vi "Get Stage Limits.vi"(0 "Notifier Names":string[](array[string]), 2 "Notifier Name":string, 7 "Stage Limits":T1[](array[typedef]), 11 "Limits Loaded?":bool) -> (4 "Limits":dbl[][](array[numeric]), 15 "Use Limits?":bool)   [LabVIEW 2016]
uses:
  Stages Limits Type Defs/Stage Limits.ctl
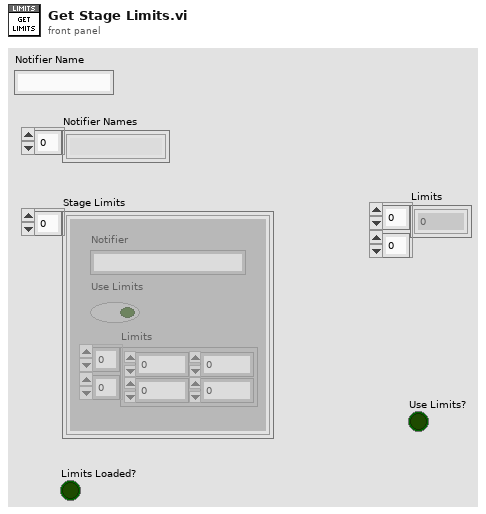
[diagram p1: front panel]
types:
  T1 = typedef "Stage Limits.ctl" = cluster{"Notifier":string, "Use Limits":bool, "Limits":dbl[][]}
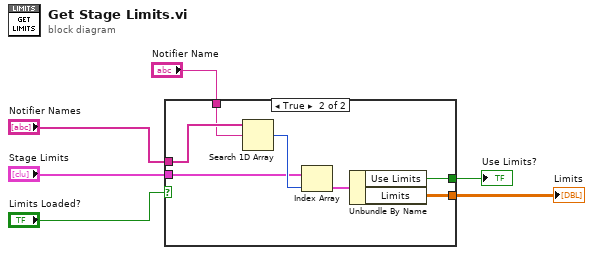
[diagram p0: block diagram]
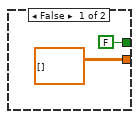
[diagram p2: hidden frame]
diagram:
  n1 = case shown="True" "Limits Loaded?" {
    tunnel: "Notifier Names" -> [_ w15]
    tunnel: "Stage Limits" -> [_ w13]
    tunnel: [dbl[][] [] ("Limits") w11] -> w1
    tunnel: [FALSE ("Use Limits") w10] -> w3
    tunnel: "Notifier Name" -> [_ w9]
    frame False {
    }
    frame True {
      n2 = Search 1D Array(1D array=w15, element=w9) -> (index of element=w14:i32)  [unwired: 1 in]
      n3 = Index Array(array=w13, index=w14) -> (element=w12:T1)
      n4 = Unbundle By Name(w12) -> ("Use Limits"=w10:bool, "Limits"=w11:dbl[][])
    }
  }
  "Use Limits?" <- w3
  "Limits" <- w1
